vi "Check Find Home.vi"(7 "Home All":bool, 8 "error in":errorcluster, 10 "Controls":T1={"Axis 1"={"Axis"=1, "Enable"=FALSE, "Start"=FALSE, "Home"=FALSE, "Stop Type"=0, "Kill"=FALSE}, "Axis 2"={"Axis"=1, "Enable"=FALSE, "Start"=FALSE, "Home"=FALSE, "Stop Type"=0, "Kill"=FALSE}, "Axis 3"={"Axis"=1, "Enable"=FALSE, "Start"=FALSE, "Home"=FALSE, "Stop Type"=0, "Kill"=FALSE}, "Axis 4"={"Axis"=1, "Enable"=FALSE, "Start"=FALSE, "Home"=FALSE, "Stop Type"=0, "Kill"=FALSE}, "Axis 5"={"Axis"=1, "Enable"=FALSE, "Start"=FALSE, "Home"=FALSE, "Stop Type"=0, "Kill"=FALSE}, "Axis 6"={"Axis"=1, "Enable"=FALSE, "Start"=FALSE, "Home"=FALSE, "Stop Type"=0, "Kill"=FALSE}} {"Axis 6"."Stop Type" items=["Decelerate", "Halt", "Kill"]; "Axis 6"."Axis" items=["Axis 1"=1, "Axis 2"=2, "Axis 3"=3, "Axis 4"=4, "Axis 5"=5, "Axis 6"=6, "Axis 7"=7, "Axis 8"=8]; "Axis 5"."Stop Type" items=["Decelerate", "Halt", "Kill"]; "Axis 5"."Axis" items=["Axis 1"=1, "Axis 2"=2, "Axis 3"=3, "Axis 4"=4, "Axis 5"=5, "Axis 6"=6, "Axis 7"=7, "Axis 8"=8]; "Axis 4"."Stop Type" items=["Decelerate", "Halt", "Kill"]; "Axis 4"."Axis" items=["Axis 1"=1, "Axis 2"=2, "Axis 3"=3, "Axis 4"=4, "Axis 5"=5, "Axis 6"=6, "Axis 7"=7, "Axis 8"=8]; "Axis 3"."Stop Type" items=["Decelerate", "Halt", "Kill"]; "Axis 3"."Axis" items=["Axis 1"=1, "Axis 2"=2, "Axis 3"=3, "Axis 4"=4, "Axis 5"=5, "Axis 6"=6, "Axis 7"=7, "Axis 8"=8]; "Axis 2"."Stop Type" items=["Decelerate", "Halt", "Kill"]; "Axis 2"."Axis" items=["Axis 1"=1, "Axis 2"=2, "Axis 3"=3, "Axis 4"=4, "Axis 5"=5, "Axis 6"=6, "Axis 7"=7, "Axis 8"=8]; "Axis 1"."Stop Type" items=["Decelerate", "Halt", "Kill"]; "Axis 1"."Axis" items=["Axis 1"=1, "Axis 2"=2, "Axis 3"=3, "Axis 4"=4, "Axis 5"=5, "Axis 6"=6, "Axis 7"=7, "Axis 8"=8]}, 11 "Bd ID In":T4) -> (0 "error out":errorcluster, 3 "Bd ID Out":T4)   [LabVIEW 2010]
doc: "Written specifically for the MultiAxisMove VI. Polls the 'Controls' cluster for a 'Home' or 'Home All' signal. If 'Home All' is true, the Find Home VI is called for all axes in parallel. Otherwise, function checks for a true 'Home' condition on each axes in parallel and calls the Find Home subVI accordingly."
uses:
  Typedefs/AxisSpaceControls_ClusterofAxisControls.ctl
  Typedefs/AxisControls_cluster.ctl
  <vilib>/Motion/FlexMotion/CustomControls/CustomControls.llb/Axis To Control.flx
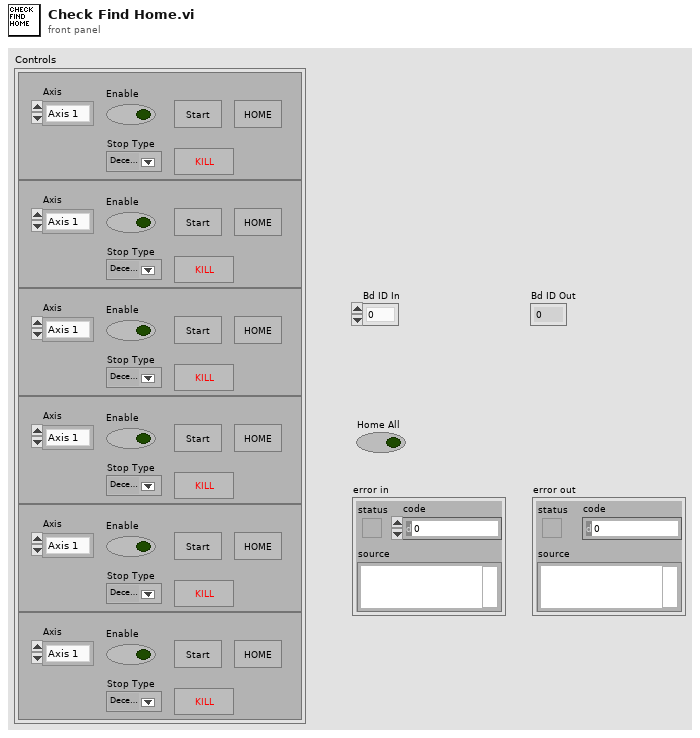
[diagram p1: front panel]
types:
  T1 = typedef "AxisSpaceControls_ClusterofAxisControls.ctl" = cluster{"Axis 1":T2, "Axis 2":T2, "Axis 3":T2, "Axis 4":T2, "Axis 5":T2, "Axis 6":T2}
  T2 = typedef "AxisControls_cluster.ctl" = cluster{"Axis":T3, "Enable":bool, "Start":bool, "Home":bool, "Stop Type":u16, "Kill":bool}
  T3 = typedef "Axis To Control.flx" = u16
  T4 = typedef "Bd Id Out" = u8
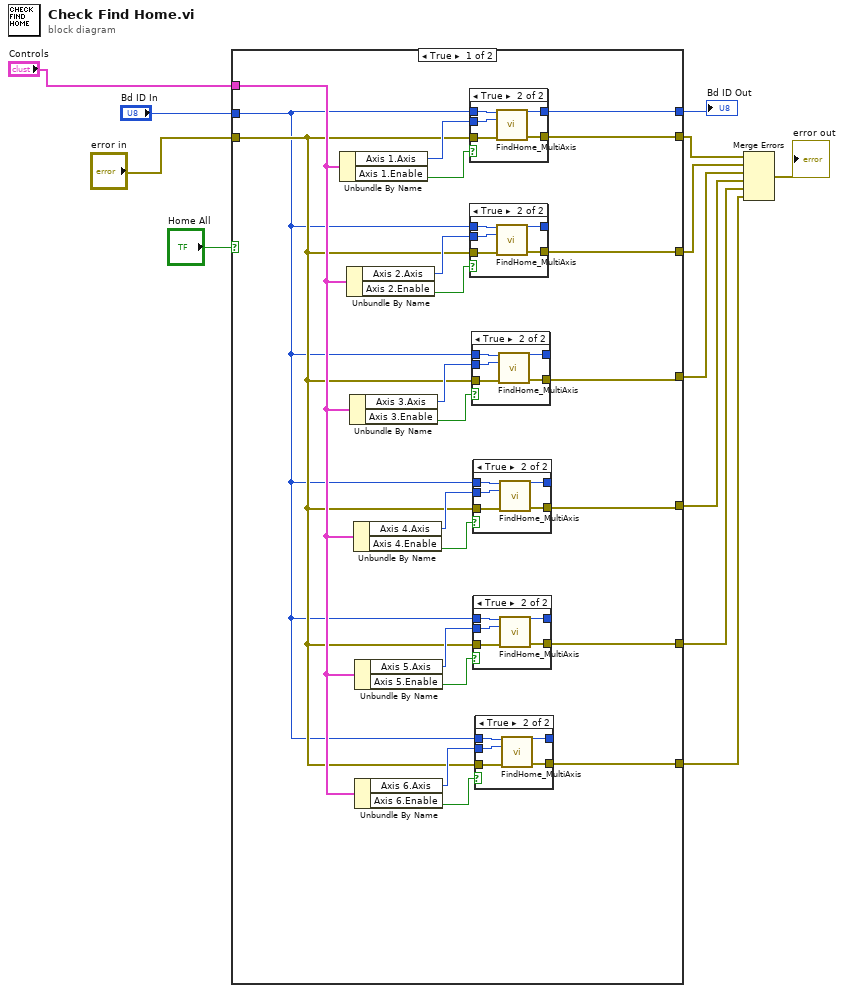
[diagram p0: block diagram]
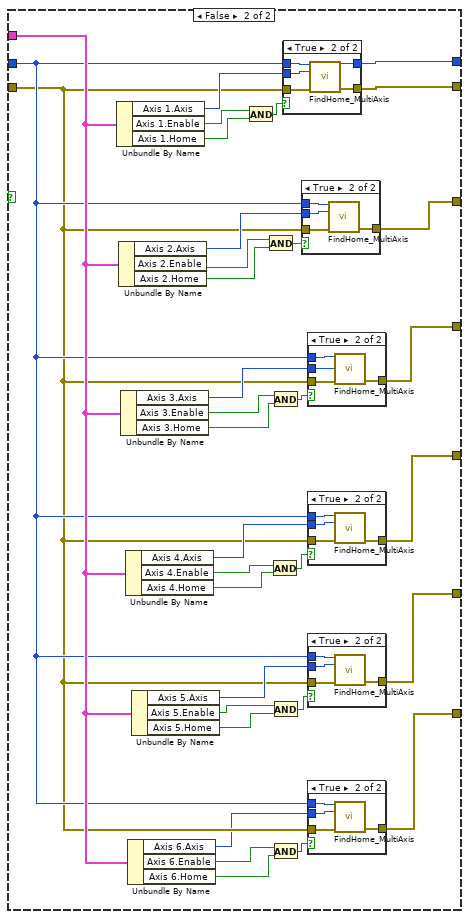
[diagram p8: hidden frame]
diagram:
  n1 = case shown="True" "Home All" {
    tunnel: "error in" -> [w26 w97]
    tunnel: "Bd ID In" -> [w19 w98]
    tunnel: "Controls" -> [w27 w108]
    tunnel: [w34 w110] -> w6
    tunnel: [w18 w107] -> w8
    tunnel: [w17 w106] -> w5
    tunnel: [w16 w102] -> w4
    tunnel: [w15 w101] -> w3
    tunnel: [w14 w99] -> w2
    tunnel: [w13 w95] -> w1
    frame True {
      n2 = Unbundle By Name(w27) -> ("Axis 1.Axis"=w33:T3, "Axis 1.Enable"=w20:bool)
      n3 = Unbundle By Name(w27) -> ("Axis 2.Axis"=w32:T3, "Axis 2.Enable"=w21:bool)
      n4 = Unbundle By Name(w27) -> ("Axis 3.Axis"=w31:T3, "Axis 3.Enable"=w22:bool)
      n5 = Unbundle By Name(w27) -> ("Axis 4.Axis"=w30:T3, "Axis 4.Enable"=w23:bool)
      n6 = Unbundle By Name(w27) -> ("Axis 5.Axis"=w29:T3, "Axis 5.Enable"=w24:bool)
      n7 = Unbundle By Name(w27) -> ("Axis 6.Axis"=w28:T3, "Axis 6.Enable"=w25:bool)
      n8 = case shown="True" w20 {
        tunnel: w26 -> [w70 w76]
        tunnel: w19 -> [w71 w75]
        tunnel: [w70 w74] -> w34
        tunnel: [w71 w73] -> w18
        tunnel: w33 -> [_ w72]
        frame False {
        }
        frame True {
          n9 = call "FindHome_MultiAxis.vi"("Bd ID In"=w75, "Axis"=w72, "error in"=w76) -> ("Bd ID Out"=w73:T4, "error out"=w74:errorcluster)  [unwired: 10 in, 1 out]
        }
      }
      n10 = case shown="True" w21 {
        tunnel: w26 -> [w63 w69]
        tunnel: w19 -> [w64 w68]
        tunnel: [w63 w67] -> w17
        tunnel: [w64 w66] -> _
        tunnel: w32 -> [_ w65]
        frame False {
        }
        frame True {
          n11 = call "FindHome_MultiAxis.vi"("Bd ID In"=w68, "Axis"=w65, "error in"=w69) -> ("Bd ID Out"=w66:T4, "error out"=w67:errorcluster)  [unwired: 10 in, 1 out]
        }
      }
      n12 = case shown="True" w22 {
        tunnel: w26 -> [w56 w62]
        tunnel: w19 -> [w57 w61]
        tunnel: [w56 w60] -> w16
        tunnel: [w57 w59] -> _
        tunnel: w31 -> [_ w58]
        frame False {
        }
        frame True {
          n13 = call "FindHome_MultiAxis.vi"("Bd ID In"=w61, "Axis"=w58, "error in"=w62) -> ("Bd ID Out"=w59:T4, "error out"=w60:errorcluster)  [unwired: 10 in, 1 out]
        }
      }
      n14 = case shown="True" w23 {
        tunnel: w26 -> [w49 w55]
        tunnel: w19 -> [w50 w54]
        tunnel: [w49 w53] -> w15
        tunnel: [w50 w52] -> _
        tunnel: w30 -> [_ w51]
        frame False {
        }
        frame True {
          n15 = call "FindHome_MultiAxis.vi"("Bd ID In"=w54, "Axis"=w51, "error in"=w55) -> ("Bd ID Out"=w52:T4, "error out"=w53:errorcluster)  [unwired: 10 in, 1 out]
        }
      }
      n16 = case shown="True" w24 {
        tunnel: w26 -> [w42 w48]
        tunnel: w19 -> [w43 w47]
        tunnel: [w42 w46] -> w14
        tunnel: [w43 w45] -> _
        tunnel: w29 -> [_ w44]
        frame False {
        }
        frame True {
          n17 = call "FindHome_MultiAxis.vi"("Bd ID In"=w47, "Axis"=w44, "error in"=w48) -> ("Bd ID Out"=w45:T4, "error out"=w46:errorcluster)  [unwired: 10 in, 1 out]
        }
      }
      n18 = case shown="True" w25 {
        tunnel: w26 -> [w35 w41]
        tunnel: w19 -> [w36 w40]
        tunnel: [w35 w39] -> w13
        tunnel: [w36 w38] -> _
        tunnel: w28 -> [_ w37]
        frame False {
        }
        frame True {
          n19 = call "FindHome_MultiAxis.vi"("Bd ID In"=w40, "Axis"=w37, "error in"=w41) -> ("Bd ID Out"=w38:T4, "error out"=w39:errorcluster)  [unwired: 10 in, 1 out]
        }
      }
    }
    frame False {
      n20 = Unbundle By Name(w108) -> ("Axis 1.Axis"=w109:T3, "Axis 1.Enable"=w92:bool, "Axis 1.Home"=w91:bool)
      n21 = Unbundle By Name(w108) -> ("Axis 2.Axis"=w104:T3, "Axis 2.Enable"=w90:bool, "Axis 2.Home"=w89:bool)
      n22 = Unbundle By Name(w108) -> ("Axis 3.Axis"=w105:T3, "Axis 3.Enable"=w87:bool, "Axis 3.Home"=w86:bool)
      n23 = Unbundle By Name(w108) -> ("Axis 4.Axis"=w103:T3, "Axis 4.Enable"=w82:bool, "Axis 4.Home"=w81:bool)
      n24 = Unbundle By Name(w108) -> ("Axis 6.Axis"=w96:T3, "Axis 6.Enable"=w78:bool, "Axis 6.Home"=w77:bool)
      n25 = Unbundle By Name(w108) -> ("Axis 5.Axis"=w100:T3, "Axis 5.Enable"=w80:bool, "Axis 5.Home"=w79:bool)
      n26 = And(x=w92, y=w91) -> (x .and. y?=w94:bool)
      n27 = And(x=w90, y=w89) -> (x .and. y?=w93:bool)
      n28 = And(x=w82, y=w81) -> (x .and. y?=w85:bool)
      n29 = And(x=w87, y=w86) -> (x .and. y?=w88:bool)
      n30 = And(x=w80, y=w79) -> (x .and. y?=w84:bool)
      n31 = And(x=w78, y=w77) -> (x .and. y?=w83:bool)
      n32 = case shown="True" w94 {
        tunnel: w97 -> [w136 w142]
        tunnel: w98 -> [w137 w141]
        tunnel: [w136 w140] -> w110
        tunnel: [w137 w139] -> w107
        tunnel: w109 -> [_ w138]
        frame False {
        }
        frame True {
          n33 = call "FindHome_MultiAxis.vi"("Bd ID In"=w141, "Axis"=w138, "error in"=w142) -> ("Bd ID Out"=w139:T4, "error out"=w140:errorcluster)  [unwired: 10 in, 1 out]
        }
      }
      n34 = case shown="True" w93 {
        tunnel: w98 -> [_ w135]
        tunnel: [w131 w134] -> w106
        tunnel: w104 -> [_ w133]
        tunnel: w97 -> [w131 w132]
        frame False {
        }
        frame True {
          n35 = call "FindHome_MultiAxis.vi"("Bd ID In"=w135, "Axis"=w133, "error in"=w132) -> ("error out"=w134:errorcluster)  [unwired: 10 in, 2 out]
        }
      }
      n36 = case shown="True" w88 {
        tunnel: [w126 w130] -> w102
        tunnel: w105 -> [_ w129]
        tunnel: w98 -> [_ w128]
        tunnel: w97 -> [w126 w127]
        frame False {
        }
        frame True {
          n37 = call "FindHome_MultiAxis.vi"("Bd ID In"=w128, "Axis"=w129, "error in"=w127) -> ("error out"=w130:errorcluster)  [unwired: 10 in, 2 out]
        }
      }
      n38 = case shown="True" w85 {
        tunnel: [w121 w125] -> w101
        tunnel: w103 -> [_ w124]
        tunnel: w97 -> [w121 w123]
        tunnel: w98 -> [_ w122]
        frame False {
        }
        frame True {
          n39 = call "FindHome_MultiAxis.vi"("Bd ID In"=w122, "Axis"=w124, "error in"=w123) -> ("error out"=w125:errorcluster)  [unwired: 10 in, 2 out]
        }
      }
      n40 = case shown="True" w84 {
        tunnel: w97 -> [w116 w120]
        tunnel: w98 -> [_ w119]
        tunnel: [w116 w118] -> w99
        tunnel: w100 -> [_ w117]
        frame False {
        }
        frame True {
          n41 = call "FindHome_MultiAxis.vi"("Bd ID In"=w119, "Axis"=w117, "error in"=w120) -> ("error out"=w118:errorcluster)  [unwired: 10 in, 2 out]
        }
      }
      n42 = case shown="True" w83 {
        tunnel: w97 -> [w111 w115]
        tunnel: w98 -> [_ w114]
        tunnel: [w111 w113] -> w95
        tunnel: w96 -> [_ w112]
        frame False {
        }
        frame True {
          n43 = call "FindHome_MultiAxis.vi"("Bd ID In"=w114, "Axis"=w112, "error in"=w115) -> ("error out"=w113:errorcluster)  [unwired: 10 in, 2 out]
        }
      }
    }
  }
  "Bd ID Out" <- w8
  n44 = Merge Errors(w6, w5, w4, w3, w2, w1) -> (→"error out":errorcluster)
